vi "Image_Handler.vi"(0 "Camera":T5, 5 "Data":T2={"L16 Linear Actuator"="", "XE 1000 Pump"="", "Camera1"="", "Camera2"="", "Img_Capt"=FALSE, "Actuator"=FALSE, "Pump"=FALSE, "Cam 1"=FALSE, "Cam 2"=FALSE, "Empty_Refill"=FALSE, "Crop"=FALSE, "Light intensity"=100, "Exposure Time"=1000.0, "Sample Name"="Test Sample", "Operator"="MRJ", "Calibration 1"=path "C:/Users/au540322/Desktop/IHS_Project/images/Debris/Debris_0/Debris_0_2019_06_01-23-32-49-686.PNG", "Calibration 2"=path "C:/Users/au540322/Desktop/IHS_Project/images/Debris/Debris_0/Debris_0_2019_06_01-23-32-49-686.PNG", "Framerate"=1, "Timeout Sample"=0, "Collection date"="MRJ", "Sample size threshold"=1, "Empty start"=1, "Command"="MRJ", "Station"="", "Species Name"="", "Other Notes"="", "Aperture"=enum."Item 0", "Image Process Queue Size"=500, "Image Save Queue Size"=500, "Overload threshold"=500, "Max Framerate"=100, "Rectangle 1"={"Left"=0, "Top"=0, "Right"=0, "Bottom"=0, "Rotation"=0.0}, "Rectangle 2"={"Left"=0, "Top"=0, "Right"=0, "Bottom"=0, "Rotation"=0.0}, "Detection Region %"=0.0, "Detect 1"=path "C:/Users/au540322/Desktop/IHS_Project/images/Debris/Debris_0/Debris_0_2019_06_01-23-32-49-686.PNG", "Detect 2"=path "C:/Users/au540322/Desktop/IHS_Project/images/Debris/Debris_0/Debris_0_2019_06_01-23-32-49-686.PNG", "Max large object threshold"=0, "Open(T)/Close(F)"=FALSE, "Img_Capt Begin"=FALSE, "Dispense Speed"=100, "Flush Size"=100, "Location"="Station", "Latitude"="Station", "Longitude"="Station", "Determiner"="Station", "Sex"="Station", "Camera1_Img"=refnum, "Camera2_Img"=refnum, "Img1_Orig_Disp"=refnum, "Img2_Orig_Disp"=refnum, "Img1_Orig_RGB"=refnum, "Img2_Orig_RGB"=refnum, "Blue_Plane_Extract"=refnum, "Subtracted_Plane"=refnum, "Img1_Binary"=refnum, "Img2_Binary"=refnum, "Crop_Mask"=refnum, "Img1_Save"=refnum, "Img2_Save"=refnum, "Img1_Cali_Full"=refnum, "Img2_Cali_Full"=refnum, "Img1_Cali_Detect"=refnum, "Img2_Cali_Detect"=refnum, "Cam 1 queue"=refnum, "Cam 1 - save queue"=refnum, "Cam 2 queue"=refnum, "Cam 2 - save queue"=refnum} {"Flush Size" min=1; "Dispense Speed" min=1; "Rectangle 2"."Rotation" format="%.2f"; "Rectangle 2"."Left" scale=0.0..1024.0; "Rectangle 2"."Right" scale=0.0..1024.0; "Rectangle 1"."Rotation" format="%.2f"; "Rectangle 1"."Left" scale=0.0..1024.0; "Rectangle 1"."Right" scale=0.0..1024.0; "Max Framerate" min=1; "Overload threshold" min=1; "Image Save Queue Size" min=1; "Image Process Queue Size" min=1; "Empty start" min=1; "Sample size threshold" min=1; "Framerate" min=1; "Light intensity" scale=0.0..100.0}, 9 "Prev. sample":i32, 11 "Timeout in":i32) -> (3 "Object":bool, 4 "Detected object":T1, 6 "Image Out":T1, 8 "Binary":T1, 10 "Sample nr":i32, 15 "Timeout out":i32)   [LabVIEW 2020]
uses:
  Camera_ID.ctl
  controls/Data.ctl
  <vilib>/userDefined/High Color/IMAQdx.ctl
  <vilib>/vision/Image Controls.llb/IMAQ Image.ctl
panel:
  out "error out 1":errorcluster
  out "error out 2":errorcluster
  in  "error in":errorcluster
  out "error out":errorcluster
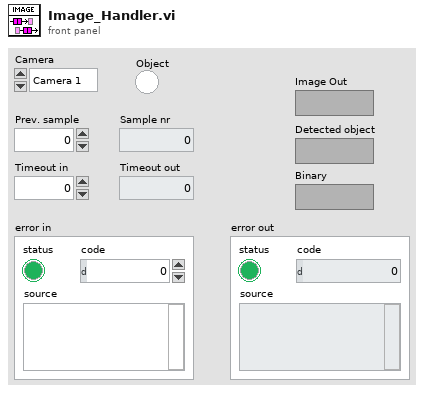
[diagram p1: front panel]
types:
  T1 = typedef "IMAQ Image.ctl" = refnum<image>
  T2 = typedef "Data.ctl" = cluster{"L16 Linear Actuator":refnum<visa-resource-name>, "XE 1000 Pump":refnum<visa-resource-name>, "Camera1":T3, "Camera2":T3, "Img_Capt":bool, "Actuator":bool, "Pump":bool, "Cam 1":bool, "Cam 2":bool, "Empty_Refill":bool, "Crop":bool, "Light intensity":i32, "Exposure Time":dbl, "Sample Name":string, "Operator":string, "Calibration 1":path, "Calibration 2":path, "Framerate":i32, "Timeout Sample":i32, "Collection date":string, "Sample size threshold":i32, "Empty start":u32, "Command":string, "Station":string, "Species Name":string, "Other Notes":string, "Aperture":enum32{"Item 0", "Item 1", "Item 2", "Item 3"}, "Image Process Queue Size":i32, "Image Save Queue Size":i32, "Overload threshold":i32, "Max Framerate":i32, "Rectangle 1":T4, "Rectangle 2":T4, "Detection Region %":dbl, "Detect 1":path, "Detect 2":path, "Max large object threshold":i32, "Open(T)/Close(F)":bool, "Img_Capt Begin":bool, "Dispense Speed":i32, "Flush Size":i32, "Location":string, "Latitude":string, "Longitude":string, "Determiner":string, "Sex":string, "Camera1_Img":T1, "Camera2_Img":T1, "Img1_Orig_Disp":T1, "Img2_Orig_Disp":T1, "Img1_Orig_RGB":T1, "Img2_Orig_RGB":T1, "Blue_Plane_Extract":T1, "Subtracted_Plane":T1, "Img1_Binary":T1, "Img2_Binary":T1, "Crop_Mask":T1, "Img1_Save":T1, "Img2_Save":T1, "Img1_Cali_Full":T1, "Img2_Cali_Full":T1, "Img1_Cali_Detect":T1, "Img2_Cali_Detect":T1, "Cam 1 queue":refnum<queue>, "Cam 1 - save queue":refnum<queue>, "Cam 2 queue":refnum<queue>, "Cam 2 - save queue":refnum<queue>}
  T3 = typedef "IMAQdx.ctl" = refnum<k21>
  T4 = typedef "IMAQ Rectangle" = cluster{"Left":i32, "Top":i32, "Right":i32, "Bottom":i32, "Rotation":dbl}
  T5 = typedef "Camera_ID.ctl" = enum16{"Camera 1", "Camera 2"}
  T6 = cluster{"Image Pixels (U32)":u32[][], "Detect Movement":bool}
  T7 = cluster{"Timestamp":string, "Image Pixels (U32)":u32[][], "Prev. sample":i32, "Sample Data":dbl[]}
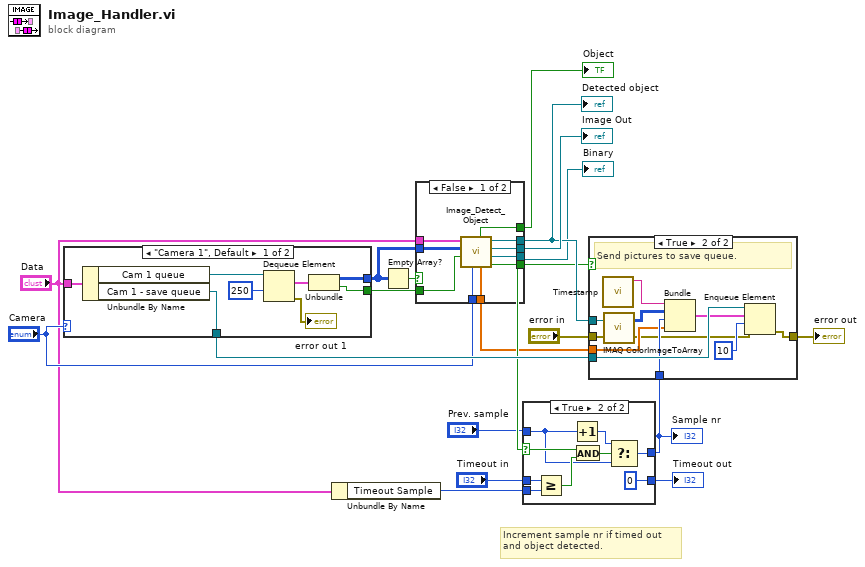
[diagram p0: block diagram]
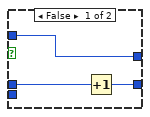
[diagram p2: hidden frame]
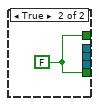
[diagram p4: hidden frame]
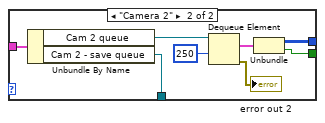
[diagram p5: hidden frame]
diagram:
  # "Increment sample nr if timed out \nand object detected."
  n1 = case shown="\"Camera 1\", Default" "Camera" {
    tunnel: "Data" -> [w27 w35]
    tunnel: [w23 w30] -> w16
    tunnel: [w22 w29] -> w7
    tunnel: [w21 w28] -> w2
    frame "Camera 1", Default {
      n2 = Unbundle By Name(w27) -> ("Cam 1 queue"=w25:refnum<queue>, "Cam 1 - save queue"=w23:refnum<queue>)
      n3 = Dequeue Element(queue=w25, timeout in ms (-1)=250) -> (element=w20:T6, error out=→"error out 1":errorcluster)  [unwired: 1 in, 2 out]
      n4 = Unbundle(w20) -> ("Image Pixels (U32)"=w22:u32[][], "Detect Movement"=w21:bool)
    }
    frame "Camera 2" {
      n5 = Unbundle By Name(w35) -> ("Cam 2 queue"=w33:refnum<queue>, "Cam 2 - save queue"=w30:refnum<queue>)
      n6 = Dequeue Element(queue=w33, timeout in ms (-1)=250) -> (element=w32:T6, error out=→"error out 2":errorcluster)  [unwired: 1 in, 2 out]
      n7 = Unbundle(w32) -> ("Image Pixels (U32)"=w29:u32[][], "Detect Movement"=w28:bool)
    }
  }
  n8 = Unbundle By Name("Data") -> ("Timeout Sample"=w9:i32)
  n9 = Empty Array?(array=w7) -> (empty?=w19:bool)
  n10 = case shown="False" w19 {
    tunnel: [w45 _] -> w17
    tunnel: [w44 w46] -> w12
    tunnel: "Data" -> [w43 _]
    tunnel: "Camera" -> [w42 _]
    tunnel: [w41 _] -> w18
    tunnel: w7 -> [w40 _]
    tunnel: [w39 _] -> w6
    tunnel: [w38 w46] -> w3
    tunnel: w2 -> [w37 _]
    tunnel: [w36 _] -> w1
    frame False {
      n11 = call "Image_Detect_Object.vi"("Camera"=w42, "Detect Crop"=w37, "Image Pixels (U32)"=w40, "Data"=w43) -> ("Object accepted"=w44:bool, "Image Binary"=w39:T1, "New image"=w41:T1, "Crop Image Out"=w45:T1, "Sample Data"=w36:dbl[], "Object"=w38:bool)  [unwired: 2 in]
    }
    frame True {
      w46 = FALSE ("Object detected")
    }
  }
  "Detected object" <- w17
  "Image Out" <- w18
  "Binary" <- w6
  "Object" <- w3
  n12 = case shown="True" w12 {
    selector: w12 -> [_ w58]
    tunnel: w9 -> [_ w57]
    tunnel: [w49 0] -> w10
    tunnel: [w48 w52] -> w8
    tunnel: "Prev. sample" -> [w48 w51]
    tunnel: "Timeout in" -> [w47 w50]
    frame False {
      n13 = Increment(x=w47) -> (x+1=w49:i32)
    }
    frame True {
      n14 = Greater Or Equal?(x=w50, y=w57) -> (x >= y?=w56:bool)
      n15 = Increment(x=w51) -> (x+1=w53:i32)
      n16 = And(x=w58, y=w56) -> (x .and. y?=w54:bool)
      n17 = Select(t=w53, s=w54, f=w51) -> (s? t:f=w52:i32)
    }
  }
  "Sample nr" <- w8
  "Timeout out" <- w10
  n18 = case shown="True" w12 {
    tunnel: w17 -> [_ w63]
    tunnel: w16 -> [_ w70]
    tunnel: "error in" -> [w59 w62]
    tunnel: [w59 w69] -> w13
    tunnel: w8 -> [_ w66]
    tunnel: w1 -> [_ w64]
    frame False {
      # "No object within criteria."
    }
    frame True {
      # "Send pictures to save queue."
      n19 = call "Timestamp.vi"() -> ("Timestamp"=w67:string)  [unwired: 11 in]
      n20 = call "IMAQ ColorImageToArray"("Image"=w63, "error in (no error)"=w62) -> ("Image Pixels (U32)"=w60:u32[][], "error out"=w61:errorcluster)  [unwired: 2 in, 1 out]
      n21 = Bundle("Timestamp"=w67, "Image Pixels (U32)"=w60, "Prev. sample"=w66, "Sample Data"=w64) -> (w68:T7)  [unwired: 1 in]
      n22 = Enqueue Element(queue=w70, element=w68, timeout in ms (-1)=10, error in (no error)=w61) -> (error out=w69:errorcluster)  [unwired: 2 out]
    }
  }
  "error out" <- w13
